vi "Restore Copy of  Cal Coefficients.vi"() -> (3 "Calibration Coefficients":T1[](array[typedef]) {"Elapsed Time" format="%<%H:%M:%S>t"; "Pump Flow Rate" format="%0d"; "Number of Zeroes" format="%0d"; "V2C" format="%0d"; "C2V" format="%0d"; "duration" format="%<%H:%M:%S>t"; "DAC" format="%03x"; "mI" format="%.3g"; "V_(RA,15mA)" format="%0.4f"; "V_(RA,5mA)" format="%0.4f"; "Chamber Temp" format="%.1f"; "Humidity" format="%.1f"})   [LabVIEW 2016]
uses:
  Controls/Calibration Coefficients.ctl
  Miscellaneous/Globals.vi
  <vilib>/Utility/file.llb/Write To Spreadsheet File (string).vi
panel:
  out "Spreadsheet":string[][](array[string])
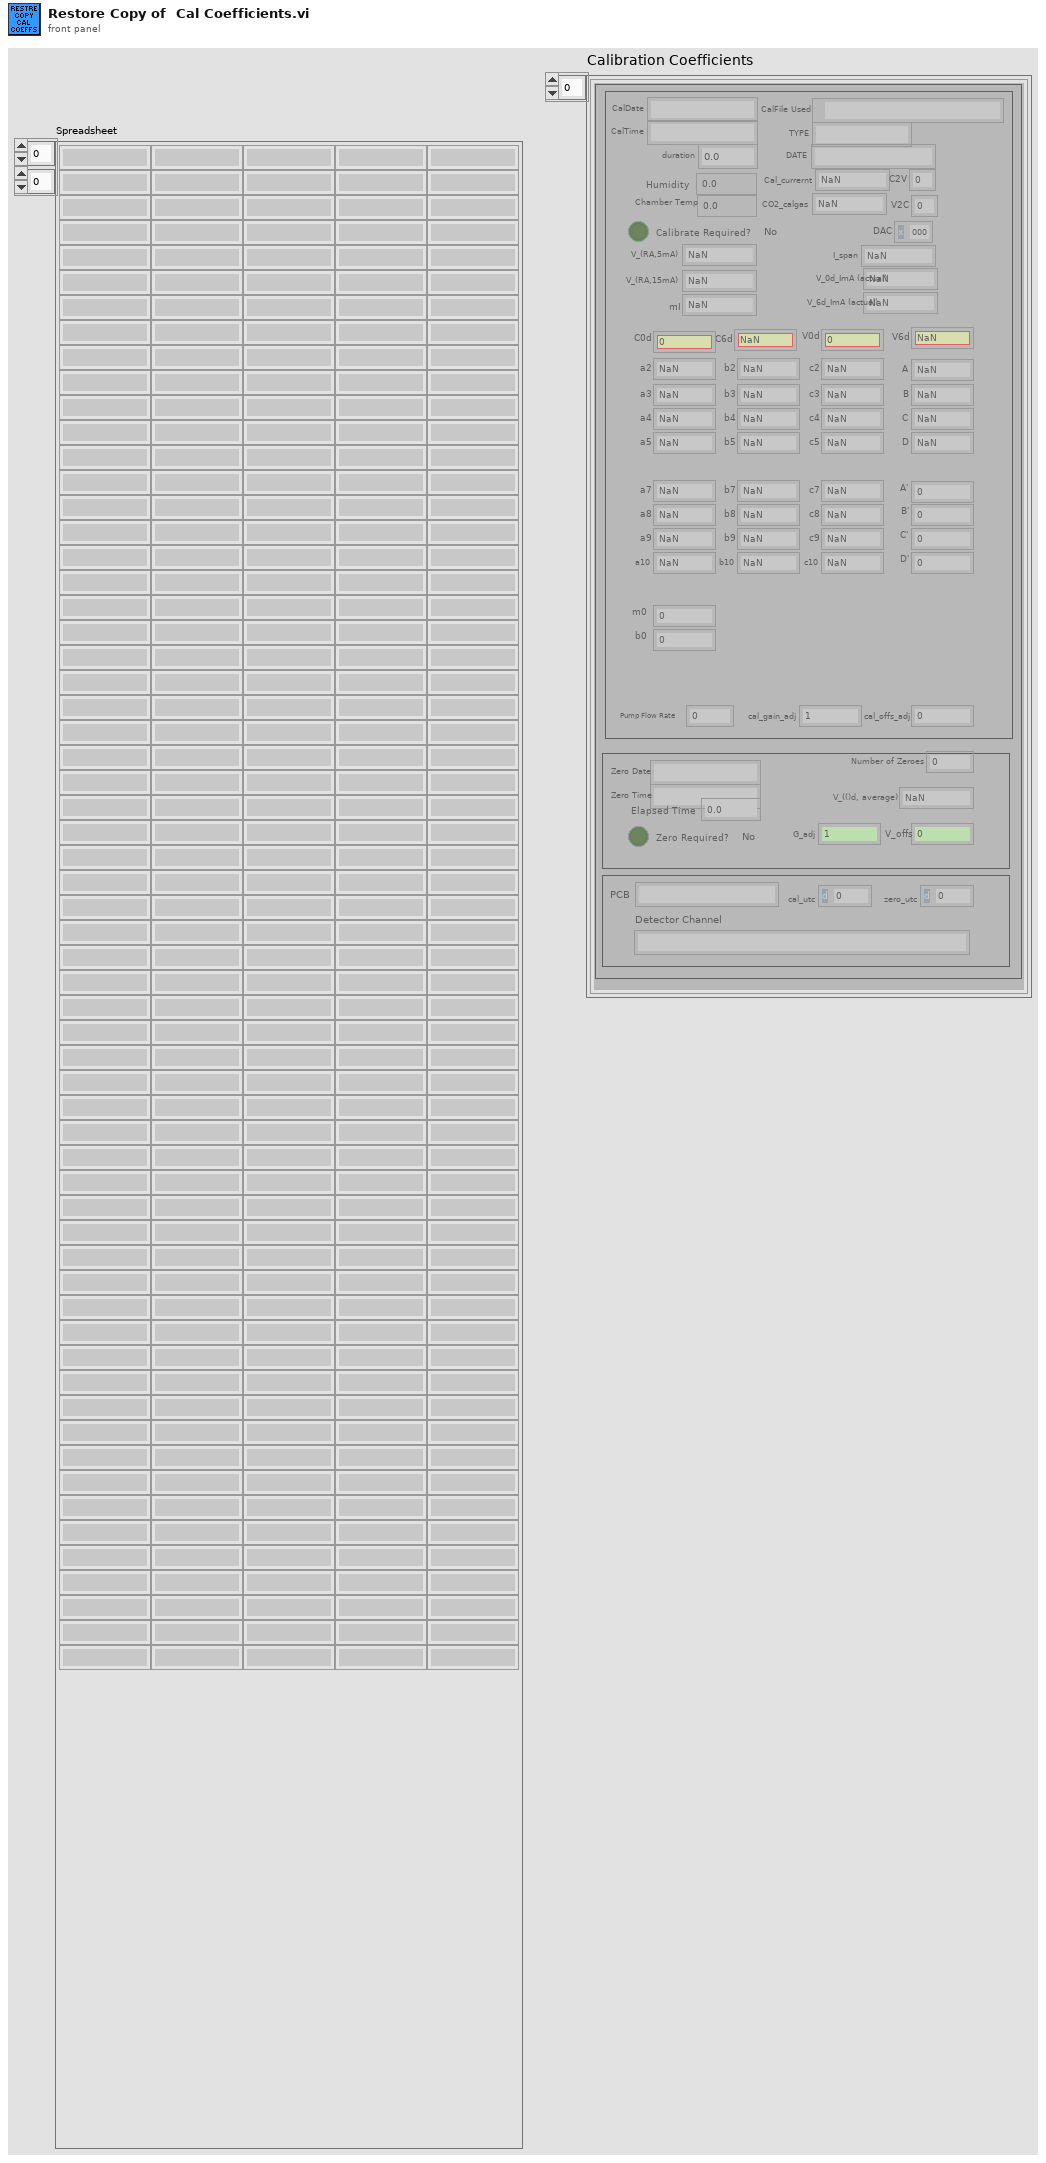
[diagram p1: front panel]
types:
  T1 = typedef "Calibration Coefficients.ctl" = cluster{"CalFile Used":path, "TYPE":string, "DATE":string, "Humidity":sgl, "Chamber Temp":dbl, "CO2_calgas":dbl, "V_(RA,5mA)":dbl, "V_(RA,15mA)":dbl, "mI":dbl, "V_0d_ImA (actual)":dbl, "V_6d_ImA (actual)":dbl, "I_span":dbl, "DAC":u16, "A":dbl, "B":dbl, "C":dbl, "D":dbl, "V6d":dbl, "A'":dbl, "B'":dbl, "C'":dbl, "D'":dbl, "V0d":dbl, "CalDate":string, "CalTime":string, "duration":dbl, "Detector Channel":string, "a2":dbl, "a3":dbl, "a4":dbl, "a5":dbl, "b2":dbl, "c2":dbl, "b3":dbl, "c3":dbl, "b4":dbl, "c4":dbl, "b5":dbl, "c5":dbl, "a7":dbl, "a8":dbl, "a9":dbl, "a10":dbl, "b7":dbl, "b8":dbl, "b9":dbl, "b10":dbl, "c7":dbl, "c8":dbl, "c9":dbl, "c10":dbl, "cal_offs_adj":dbl, "cal_gain_adj":dbl, "C6d":dbl, "C0d":dbl, "Cal_currernt":dbl, "C2V":u16, "V2C":u16, "Zero Date":string, "Zero Time":string, "Number of Zeroes":u16, "V_(()d, average)":dbl, "V_offs ":dbl, "G_adj":dbl, "Pump Flow Rate":u16, "Zero Required? ":bool, "Calibrate Required?":bool, "cal_utc":dbl, "zero_utc":dbl, "Elapsed Time":dbl, "PCB":string, "m0":dbl, "b0":dbl}
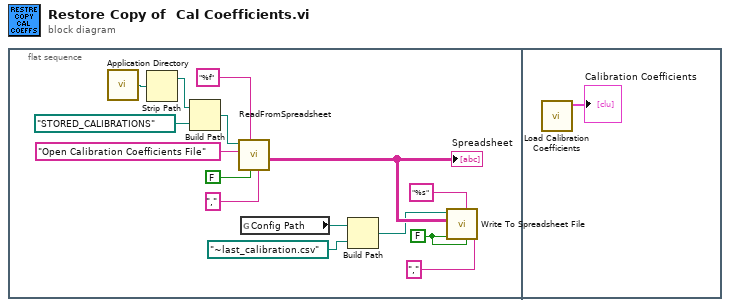
[diagram p0: block diagram]
diagram:
  n1 = flat-sequence {
    frame #0 {
      w14 = FALSE ("transpose (no:F)")
      n2 = call <vilib>:"Application Directory.vi"() -> ("Application Directory"=w3:path)
      n3 = Strip Path(path=w3) -> (stripped path=w2:path)  [unwired: 1 out]
      n4 = Build Path(base path=w2, name or relative path=path "STORED_CALIBRATIONS" ("Calfile")) -> (appended path=w1:path)
      n5 = call "ReadFromSpreadsheet.vi"("delimiter (\\t)"="," ("delimiter (\\t)"), "transpose (no:F)"=FALSE, "format (%d)"="%f", "File Prompt"="Open Calibration Coefficients File", "file path"=w1) -> ("text array"=w9:string[][])  [unwired: 2 in, 4 out]
      "Spreadsheet" <- w9
      n6 = global read "Globals.vi" "Config Path"() -> (w6:path)
      n7 = Build Path(base path=w6, name or relative path=path "~last_calibration.csv" ("Calfile")) -> (appended path=w8:path)
      n8 = call-poly <vilib>:"Write To Spreadsheet File.vi"("delimiter (\\t)"="," ("delimiter (\\t)"), "transpose? (no:F)"=w14, "format (%s)"="%s" ("format (%d)"), "append to file? (new file:F)"=w14, "2D data"=w9, "file path (dialog if empty)"=w8) -> ()  [unwired: 2 in, 1 out]
    }
    frame #1 {
      n9 = call "Load Calibration Coefficients.vi"() -> ("Calibration Coefficients"=→"Calibration Coefficients":T1[])  [unwired: 11 in]
    }
  }
